vi "Load Config.vi"(6 "Constants":refnum<class "Sequence Constants.lvclass">, 8 "error in (no error)":refnum<class "MultiErrors.lvclass">, 10 "Config Element":refnum<class "Config Element.lvclass">, 11 "Digital Command Config in":refnum<class "Digital Command Config.lvclass">) -> (0 "error out":refnum<class "MultiErrors.lvclass">, 3 "Digital Command Config out":refnum<class "Digital Command Config.lvclass">)   [LabVIEW 2020, in "VolatusSeqConfig.lvlib" / "Digital Command Config.lvclass"]
uses:
  Digital Command Config.lvclass
  VolatusErrorUtilities/MultiErrors/MultiErrors.lvclass
  lv-cdm/CDM-Config/Config Element/Config Element.lvclass
  Digital Command Config.lvclass/Digital Command Config.ctl
  Sequence Constants/Sequence Constants.lvclass
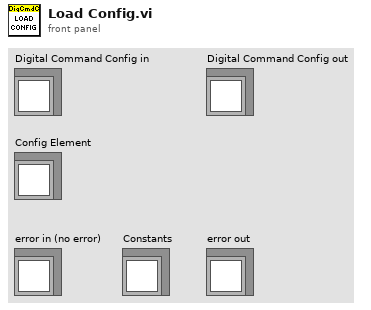
[diagram p1: front panel]
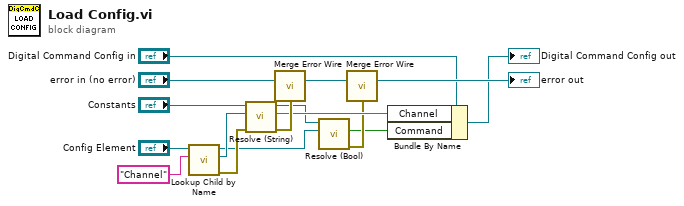
[diagram p0: block diagram]
diagram:
  n1 = call "Lookup Child by Name.vi"("Name"="Channel", "Config Element in"="Config Element") -> ("error out"=w8:errorcluster, "Child"=w9:refnum<class "Config Element.lvclass">, "Config Element out"=w2:refnum<class "Config Element.lvclass">)  [unwired: 6 in, 1 out]
  n2 = call "Resolve (String).vi"("error in (no error)"=w8, "Element"=w9, "Sequence Constants in"="Constants") -> ("error out"=w7:errorcluster, "String Value"=w6:string, "Sequence Constants out"=w1:refnum<class "Sequence Constants.lvclass">)  [unwired: 6 in]
  n3 = call "Merge Error Wire.vi"("error in (no error)"=w7, "MultiErrors in"="error in (no error)") -> ("MultiErrors out"=w10:refnum<class "MultiErrors.lvclass">)  [unwired: 13 in]
  n4 = call "Resolve (Bool).vi"("Element"=w2, "Sequence Constants in"=w1) -> ("error out"=w4:errorcluster, "Bool Value"=w3:bool)  [unwired: 7 in, 1 out]
  n5 = call "Merge Error Wire.vi"("error in (no error)"=w4, "MultiErrors in"=w10) -> ("MultiErrors out"=→"error out":refnum<class "MultiErrors.lvclass">)  [unwired: 13 in]
  n6 = Bundle By Name(cluster="Digital Command Config in", "Channel"=w6, "Command"=w3) -> (→"Digital Command Config out":refnum<class "Digital Command Config.lvclass">)
